vi "Agilent 532XX Series Acquire Multiple Frequency.vi"() -> ()   [LabVIEW 2021]
doc: "This example shows how to acquire multiple frequency using the VIs of the driver."
uses:
  <instrlib>/Agilent 532XX Series/Public/Configure/Measurement/Configure Measurement (Frequency).vi
  <instrlib>/Agilent 532XX Series/Public/Data/Read Measurement (Multiple).vi
  <instrlib>/Agilent 532XX Series/Agilent 532XX Series.lvlib
panel:
  in  "Frequency Resolution (1 Hz)":dbl=1.0
  in  "Frequency Estimate (10E+6 Hz)":dbl=10000000.0 format="%^#_6g"
  in  "Channel (1:Channel 1)":i32(ring)=1 items=["Channel 1"=1, "Channel 2"=2, "Channel 3"=3]
  in  "Number of Measurement (10)":u32=10
  out "Frequency":dbl[](array[numeric]) format="%#_12g"
  in  "Timeout (10000 ms)":u32=10000
  in  "VISA resource name":refnum<visa-resource-name>
  # "(c) 2010-2015 National Instruments.  ALL RIGHTS RESERVED."
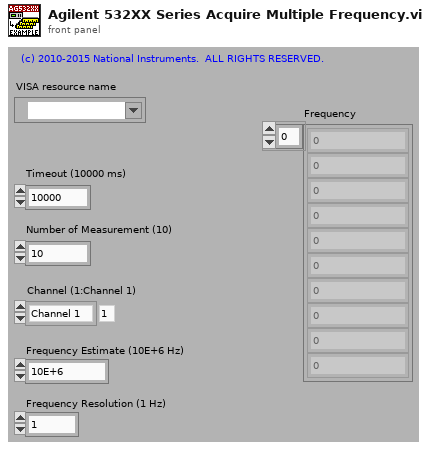
[diagram p1: front panel]
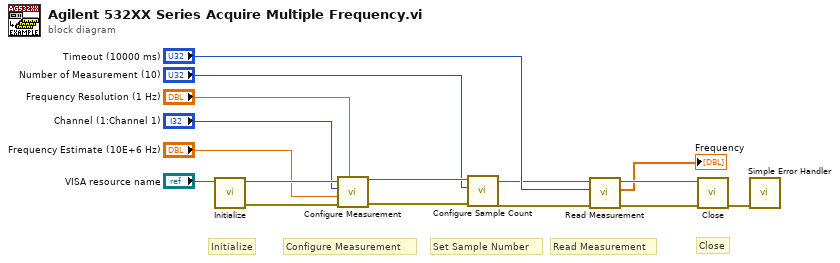
[diagram p0: block diagram]
diagram:
  # "Set Sample Number"
  # "Close"
  # "Read Measurement"
  # "Initialize"
  # "Configure Measurement"
  n1 = call <instrlib>:"Initialize.vi"("VISA resource name"="VISA resource name") -> ("error out"=w6:errorcluster, "VISA resource name out"=w5:refnum<visa-resource-name>)  [unwired: 3 in, 6 out]
  n2 = call-poly <instrlib>:"Configure Measurement.vi"("Frequency Resolution (1 Hz)"="Frequency Resolution (1 Hz)", "error in (no error)"=w6, "Frequency Estimate (10E+6 Hz)"="Frequency Estimate (10E+6 Hz)", "Channel (1:Channel 1)"="Channel (1:Channel 1)", "VISA resource name"=w5) -> ("error out"=w7:errorcluster, "VISA resource name out"=w8:refnum<visa-resource-name>)  [unwired: 5 out]
  n3 = call <instrlib>:"Configure Sample Count.vi"("error in (no error)"=w7, "Sample Count (1)"="Number of Measurement (10)", "VISA resource name"=w8) -> ("error out"=w10:errorcluster, "VISA resource name out"=w9:refnum<visa-resource-name>)  [unwired: 7 out]
  n4 = call-poly <instrlib>:"Read Measurement.vi"("error in (no error)"=w10, "Timeout (10000 ms)"="Timeout (10000 ms)", "VISA resource name"=w9) -> ("error out"=w13:errorcluster, "Measurements"=→"Frequency":dbl[], "VISA resource name out"=w12:refnum<visa-resource-name>)  [unwired: 6 out]
  n5 = call <instrlib>:"Close.vi"("error in (no error)"=w13, "VISA resource name"=w12) -> ("error out"=w15:errorcluster)  [unwired: 9 out]
  n6 = call <vilib>:"Simple Error Handler.vi"("error in (no error)"=w15) -> ()  [unwired: 1 in, 8 out]
